vi "Synchronous Read.vi"(8 "error in":errorcluster, 11 "Serial Session in":refnum<class "Serial Session.lvclass">) -> (0 "error out":errorcluster, 2 "Data Out":string, 3 "Serial Session out":refnum<class "Serial Session.lvclass">)   [LabVIEW 2015, in "Serial Session.lvclass"]
doc: "Returns data from a serial device based on a synchrnous read.\n\nHow this VI reads from the port is depending on how it is configured. If the read terminates on a character, then we simply request a read. If there is no termination charcater then we will wait for bytes based on the properties <b>Timeout (ms)</b> and <b>Loop Time (ms)</b>. In this latter case, we will read from the port based on checking the port regularly, based on the <b>Loop Time (ms)</b> property. The loop will complete after n = <b>Timeout (ms)/Loop Time (ms)</b> times or if there are no bytes on the port.\n\nThe output data string is trimmed to remove any leading or proceceding whitespace."
uses:
  Serial Session.lvclass
  Serial Session.lvclass/Serial Session.ctl
  <vilib>/Platform/TimedLoop/XDataNode/timing_clust.ctl
  <vilib>/Platform/TimedLoop/XDataNode/nitl_modes.ctl
  <vilib>/Platform/TimedLoop/XDataNode/wakeup.ctl
  <vilib>/Platform/TimedLoop/XDataNode/XDataNode.xnode
  <vilib>/Platform/TimedLoop/XDataNode/XDNodeRunTimeDep.lvlib
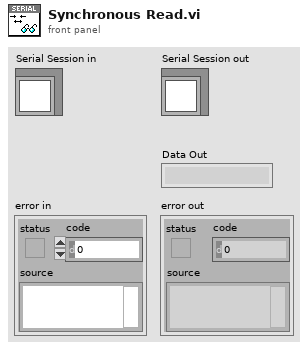
[diagram p1: front panel]
types:
  T1 = typedef "XDNodeRunTimeDep.lvlib/timing_clust.ctl" = cluster{"Expected End [f-1]":u64, "Actual End [f-1]":u64, "Finished Late? [f-1]":bool, "Expected End [i-1]":u64, "Actual End [i-1]":u64, "Finished Late? [i-1]":bool, "Expected Start [i]":u64, "Actual Start [i]":u64, "Expected Start [f]":u64, "Actual Start [f]":u64, "Source Name":string, "Structure Name":string, "Period":i64, "Deadline":i64, "Offset":i64, "Start":i64, "Priority":i32, "Timeout":i32, "Mode":T2, "Wakeup Reason":T3, "Error":errorcluster, "Source Type":string, "Secondary Source Type":string, "Global End Time":u64, "Global Start Time":u64, "Frame Duration":u64, "Iteration Duration":u64, "Assigned CPU":i32, "I/O Scan Engine Mode":u32}
  T2 = typedef "XDNodeRunTimeDep.lvlib/nitl_modes.ctl" = enum32{"No Change", "Process missed periods, maintain original phase", "Discard missed periods, maintain original phase", "Process missed periods, ignore original phase", "Discard missed periods, ignore original phase"}
  T3 = typedef "XDNodeRunTimeDep.lvlib/wakeup.ctl" = enum32{"Normal", "Aborted", "Asynchronous wakeup", "Timing source error", "Timed loop error", "Timeout"}
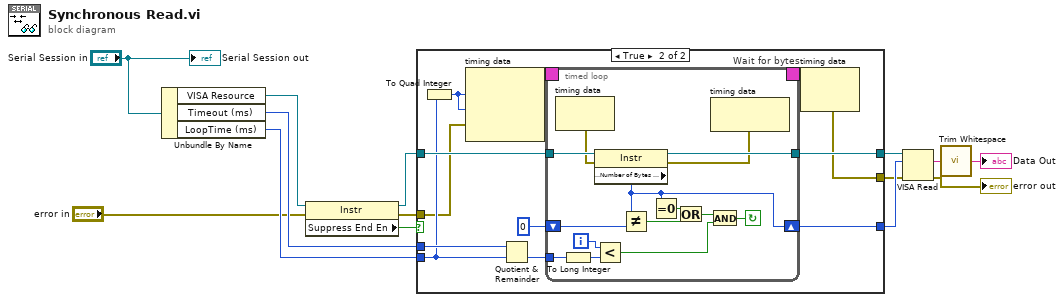
[diagram p0: block diagram]
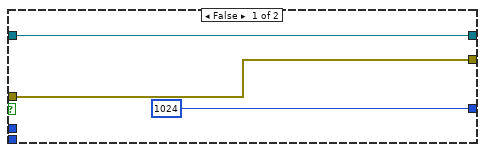
[diagram p2: hidden frame]
diagram:
  n1 = Unbundle By Name("Serial Session in") -> ("VISA Resource"=w14:refnum<visa-resource-name>, "Timeout (ms)"=w10:u32, "LoopTime (ms)"=w9:u32)
  n2 = property class="Instr"(reference=w14, error in="error in") -> (reference out=w11:refnum<visa-resource-name>, error out=w12:errorcluster, "Suppress End En"=w13:bool)
  n3 = case shown="True" w13 {
    tunnel: w11 -> [w16 w27]
    tunnel: [w16 w26] -> w7
    tunnel: [u32 1024 w25] -> w6
    tunnel: w10 -> [_ w24]
    tunnel: w9 -> [_ w23]
    tunnel: w12 -> [w17 w22]
    tunnel: [w17 w21] -> w5
    frame False {
    }
    frame True {
      n4 = To Quad Integer(1:w23) -> (0:w18:i64)
      n5 = node-c288(w18, w18, w22) -> (w29:T1)
      n6 = Quotient & Remainder(x=w24, y=w23) -> (floor(x/y)=w20:u32)  [unwired: 1 out]
      n7 = timed-loop "Wait for bytes" {
        tunnel: w27 -> [w43]
        tunnel: [w42] -> w26
        tunnel: w20 -> [w31]
        shift-right: [w34] -> w25
        shift-left: u32 0 -> [w35]
        timing: w29 -> [_]
        timing-out: [_] -> w28
        i -> [w41]
        stop <- w40 continue-if-true
        n8 = node-c288() -> (w33:errorcluster)  [unwired: 1 in]
        n9 = To Long Integer(number=w31) -> (32bit integer=w30:i32)
        n10 = property class="Instr"(reference=w43, error in=w33) -> (reference out=w42:refnum<visa-resource-name>, error out=w32:errorcluster, "Serial Settings:Number of Bytes at Serial Port"=w34:u32)
        n11 = Less?(x=w41, y=w30) -> (x < y?=w39:bool)
        n12 = Not Equal?(x=w34, y=w35) -> (x != y?=w38:bool)
        n13 = Equal To 0?(x=w34) -> (x = 0?=w37:bool)
        n14 = Or(x=w37, y=w38) -> (x .or. y?=w36:bool)
        n15 = And(x=w36, y=w39) -> (x .and. y?=w40:bool)
        n16 = node-c288(w32) -> ()  [unwired: 1 out]
      }
      n17 = node-c288(w28) -> (w21:errorcluster)
    }
  }
  n18 = VISA Read(VISA resource name=w7, byte count=w6, error in (no error)=w5) -> (read buffer=w8:string, error out=→"error out":errorcluster)  [unwired: 2 out]
  n19 = call <vilib>:"Trim Whitespace.vi"("string"=w8) -> ("trimmed string"=→"Data Out":string)  [unwired: 1 in]
  "Serial Session out" <- "Serial Session in"
